vi "Build XML Filename.vi"(9 "Xml Filename In":string, 10 "SubFolder In":string, 11 "Folder In":string) -> (1 "ok?":bool, 3 "Full Filename Out":path)   [LabVIEW 2026]
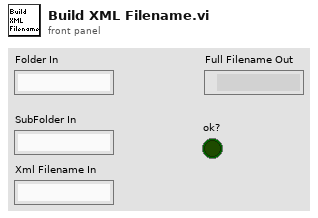
[diagram p1: front panel]
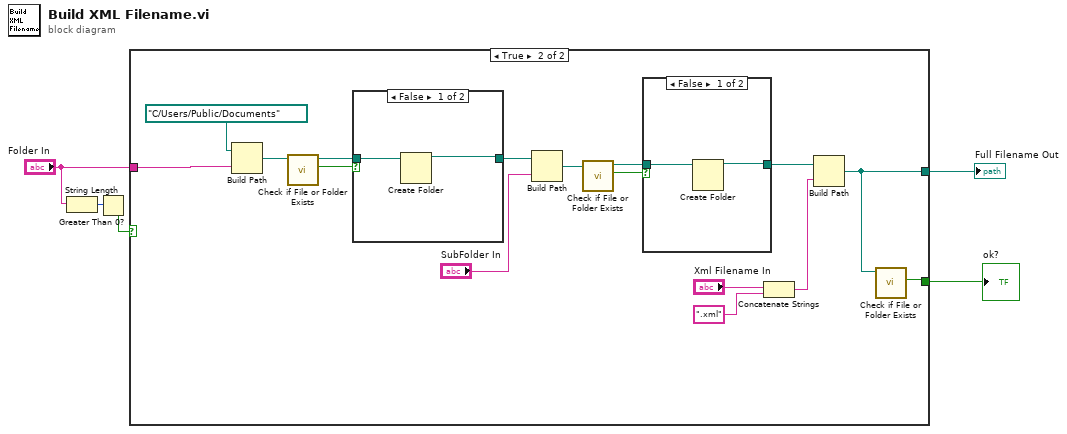
[diagram p0: block diagram]
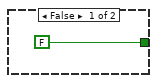
[diagram p2: hidden frame]
diagram:
  n1 = String Length(string="Folder In") -> (length=w3:i32)
  n2 = Greater Than 0?(x=w3) -> (x > 0?=w2:bool)
  n3 = case shown="True" w2 {
    tunnel: "Folder In" -> [_ w21]
    tunnel: [_ w7] -> w5
    tunnel: [FALSE w8] -> w1
    frame False {
    }
    frame True {
      n4 = Build Path(base path=path "C:/Users/Public/Documents", name or relative path=w21) -> (appended path=w20:path)
      n5 = call <vilib>:"Check if File or Folder Exists.vi"("path"=w20) -> ("file or folder exists?"=w19:bool, "dup path"=w18:path)  [unwired: 8 in, 1 out]
      n6 = case shown="False" w19 {
        tunnel: w18 -> [w27 w28]
        tunnel: [w26 w28] -> w17
        frame False {
          n7 = Create Folder(path (use dialog)=w27) -> (created path=w26:path)  [unwired: 2 in, 2 out]
        }
        frame True {
        }
      }
      n8 = Build Path(base path=w17, name or relative path="SubFolder In") -> (appended path=w15:path)
      n9 = call <vilib>:"Check if File or Folder Exists.vi"("path"=w15) -> ("file or folder exists?"=w14:bool, "dup path"=w13:path)  [unwired: 8 in, 1 out]
      n10 = case shown="False" w14 {
        tunnel: w13 -> [w24 w25]
        tunnel: [w23 w25] -> w12
        frame False {
          n11 = Create Folder(path (use dialog)=w24) -> (created path=w23:path)  [unwired: 2 in, 2 out]
        }
        frame True {
        }
      }
      n12 = Concatenate Strings("Xml Filename In", ".xml") -> (w9:string)
      n13 = Build Path(base path=w12, name or relative path=w9) -> (appended path=w7:path)
      n14 = call <vilib>:"Check if File or Folder Exists.vi"("path"=w7) -> ("file or folder exists?"=w8:bool)  [unwired: 8 in, 2 out]
    }
  }
  "Full Filename Out" <- w5
  "ok?" <- w1
